vi "get array.vi"(8 "error in (no error)":errorcluster, 10 "y array in":i32[](array[numeric]), 11 "x array in":i32[](array[numeric])) -> (0 "error out":errorcluster, 2 "y out array":i32[](array[numeric]), 3 "x out array":i32[](array[numeric]))   [LabVIEW 2016]
doc: "This vi takes a x and y array and makes sure that each point has at least 1 y value attached to it"
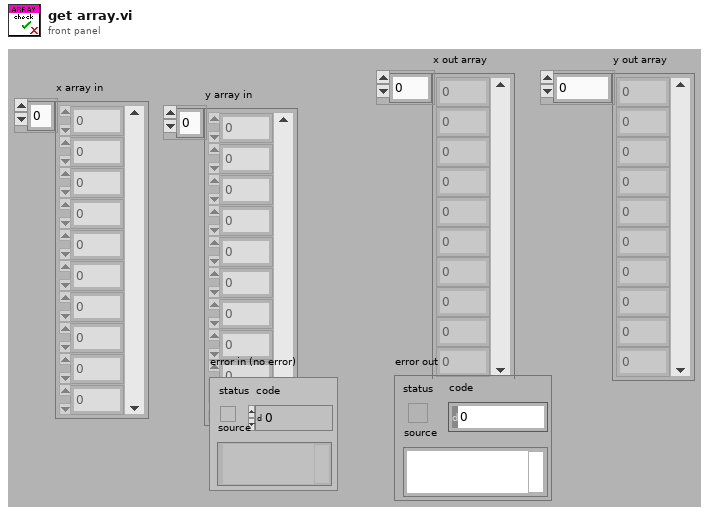
[diagram p1: front panel]
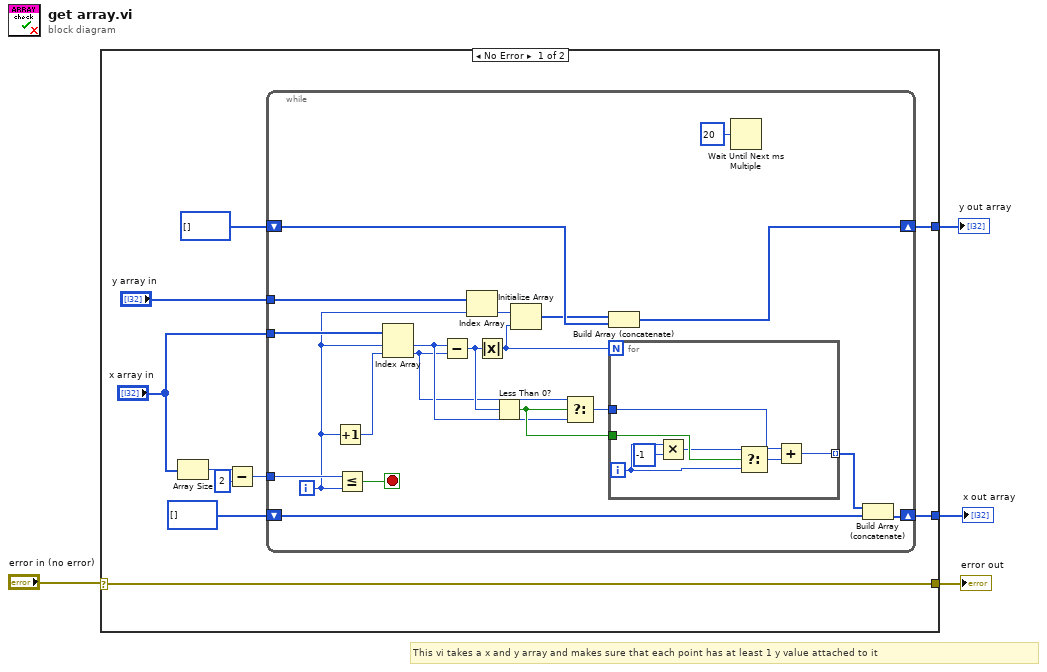
[diagram p0: block diagram]
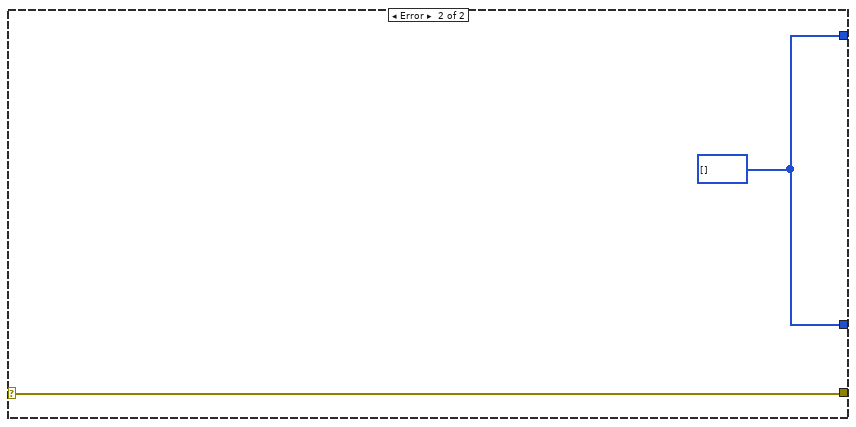
[diagram p2: hidden frame]
diagram:
  # "This vi takes a x and y array and makes sure that each point has at least 1 y value attached to it"
  n1 = case shown="No Error" "error in (no error)" {
    selector: "error in (no error)" -> [w5 w42]
    tunnel: [w12 w43] -> w4
    tunnel: [w11 w43] -> w3
    tunnel: [w5 w42] -> w1
    frame No Error {
      n2 = Array Size(array="x array in") -> (size(s)=w9:i32)
      n3 = Subtract(x=w9, y=2) -> (x-y=w10:i32)
      n4 = while {
        tunnel: "x array in" -> [w33]
        tunnel: "y array in" -> [w30]
        shift-right: [w28] -> w12
        shift-left: i32[] [] -> [w19]
        tunnel: w10 -> [w32]
        shift-right: [w17] -> w11
        shift-left: i32[] [] -> [w26]
        i -> [w15]
        stop <- w34 stop-if-true
        n5 = Increment(x=w15) -> (x+1=w31:i32)
        n6 = Less Or Equal?(x=w32, y=w15) -> (x <= y?=w34:bool)
        n7 = Index Array(array=w33, index #1=w15, index #2=w31) -> (element #1=w23:i32, element #2=w16:i32)
        n8 = Subtract(x=w23, y=w16) -> (x-y=w22:i32)
        n9 = Index Array(array=w30, index=w15) -> (element=w29:i32)
        n10 = Absolute Value(x=w22) -> (abs(x)=w20:i32)
        n11 = Less Than 0?(x=w22) -> (x < 0?=w25:bool)
        n12 = Initialize Array(w29, w20) -> (w18:i32[])
        n13 = Select(t=w16, s=w25, f=w23) -> (s? t:f=w24:i32)
        n14 = Build Array (concatenate)(w18, w19) -> (w28:i32[])
        n15 = for {
          N: w20 -> [_]
          tunnel: w24 -> [w41]
          tunnel: [w37] -> w27 mode=indexing
          tunnel: w25 -> [w38]
          i -> [w36]
          n16 = Multiply(x=w36, y=-1) -> (x*y=w35:i32)
          n17 = Select(t=w35, s=w38, f=w36) -> (s? t:f=w39:i32)
          n18 = Add(x=w41, y=w39) -> (x+y=w37:i32)
        }
        n19 = Wait Until Next ms Multiple(millisecond multiple=u32 20) -> ()  [unwired: 1 out]
        n20 = Build Array (concatenate)(w27, w26) -> (w17:i32[])
      }
    }
    frame Error {
      w43 = i32[] []
    }
  }
  "y out array" <- w4
  "x out array" <- w3
  "error out" <- w1
